vi "StartPeriodicTrigger.vi"(8 "error in (no error)":errorcluster, 10 "time (ms)":i32, 11 "Triggerable":refnum<class "Triggerable.lvclass">) -> (0 "error out":errorcluster, 3 "TriggerID":u32)   [LabVIEW 2020, in "PeriodicTrigger.lvlib"]
uses:
  PeriodicTrigger.lvlib
  Triggerable_interface/Triggerable.lvclass
  PeriodicTriggerProcess.vi
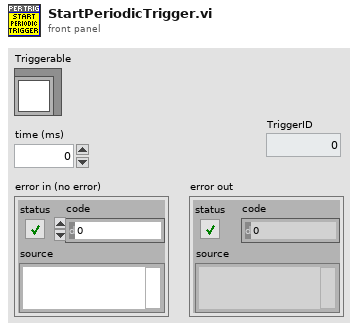
[diagram p1: front panel]
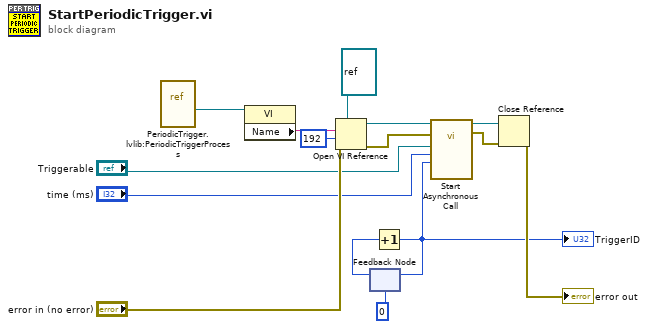
[diagram p0: block diagram]
diagram:
  n1 = vi-ref "PeriodicTrigger.lvlib:PeriodicTriggerProcess.vi"() -> (w15:refnum<vi>)
  n2 = property class="VI"(reference=w15) -> ("Name"=w14:string)  [unwired: 1 in, 2 out]
  n3 = Open VI Reference(type specifier VI Refnum (for type only)=refnum<vi> refnum, vi path=w14, options=192, error in (no error)="error in (no error)") -> (vi reference=w11:refnum<vi>, error out=w10:errorcluster)  [unwired: 2 in]
  n4 = feedback #1(u32 0) -> (w3:u32)
  n5 = Increment(x=w3) -> (x+1=w1:u32)
  "TriggerID" <- w1
  n6 = feedback-in #1(w1) -> ()
  n7 = call-by-ref "Start Asynchronous Call"(reference=w11, error in=w10, "ID"=w1, "time (ms)"="time (ms)", "Triggerable"="Triggerable") -> (reference out=w9:refnum<vi>, error out=w8:errorcluster)  [unwired: 9 in]
  n8 = Close Reference(reference=w9, error in (no error)=w8) -> (error out=→"error out":errorcluster)
